vi "Update Cell Value.vi"(8 "error in":errorcluster, 9 "Value":string, 10 "cell position in":T1, 11 "MulticolumnListbox in":refnum<vi>) -> (0 "error out":errorcluster, 3 "MulticolumnListbox out":refnum<vi>)   [LabVIEW 2014, in "Table Manager.lvlib" / "Multi Column Listbox.lvclass"]
uses:
  Multi Column Listbox.lvclass
  <vilib>/Utility/miscctls.llb/LVRowAndColumnTypeDef.ctl
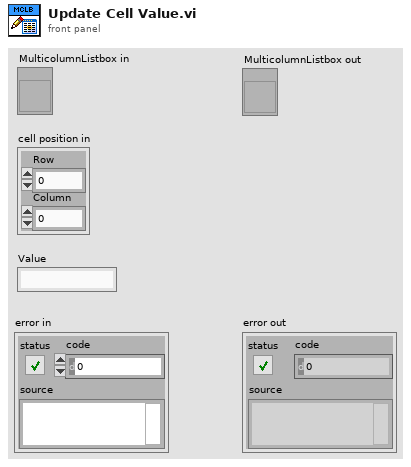
[diagram p1: front panel]
types:
  T1 = typedef "LVRowAndColumnTypeDef.ctl" = cluster{"Row":i32, "Column":i32}
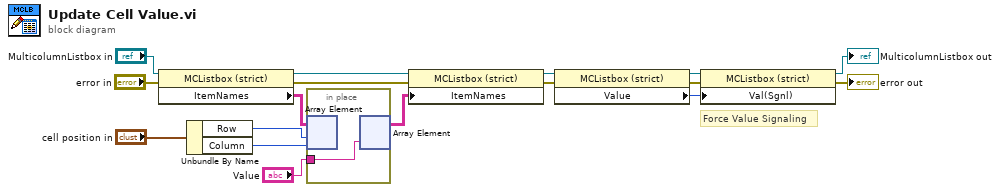
[diagram p0: block diagram]
diagram:
  # "Force Value Signaling"
  n1 = property class="MCListbox (strict)"(reference="MulticolumnListbox in", error in="error in") -> (reference out=w8:refnum<vi>, error out=w10:errorcluster, "ItemNames"=w16:string[][])
  n2 = Unbundle By Name("cell position in") -> ("Row"=w13:i32, "Column"=w12:i32)
  n3 = in-place {
    in-place-border: "Value" -> [w18]
    n4 = in-place-array #1(w16, w13, w12) -> ()  [unwired: 1 out]
    n5 = in-place-array #1(w18) -> (w15:string[][])  [unwired: 2 out]
  }
  n6 = property class="MCListbox (strict)"(reference=w8, error in=w10, "ItemNames"=w15) -> (reference out=w5:refnum<vi>, error out=w3:errorcluster)
  n7 = property class="MCListbox (strict)"(reference=w5, error in=w3) -> (reference out=w7:refnum<vi>, error out=w6:errorcluster, "Value"=w1:i32)
  n8 = property class="MCListbox (strict)"(reference=w7, error in=w6, "Val(Sgnl)"=w1) -> (reference out=→"MulticolumnListbox out":refnum<vi>, error out=→"error out":errorcluster)
